vi "format Impedance display.vi"(11 "Imp Value":dbl format="%#_13g") -> (3 "decimal integer string":string)   [LabVIEW 2016, in "CML UI.lvlib"]
doc: "<b>Note:</b> This VI was modified by the <b>Validate DQMH Module</b> tool to turn off automatic error handling."
uses:
  CML UI.lvlib
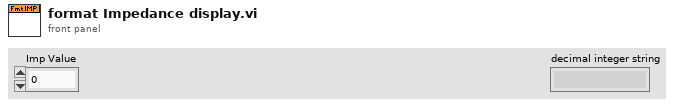
[diagram p1: front panel]
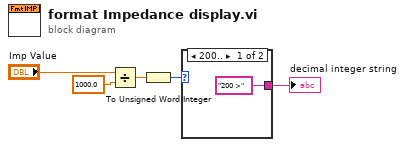
[diagram p0: block diagram]
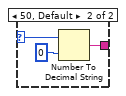
[diagram p2: hidden frame]
diagram:
  n1 = Divide(x="Imp Value", y=1000.0) -> (x/y=w3:dbl)
  n2 = To Unsigned Word Integer(number=w3) -> (unsigned 16bit integer=w2:u16)
  n3 = case shown="200.." w2 {
    selector: w2 -> [_ w8]
    tunnel: ["200 >" w7] -> w1
    frame 200.. {
    }
    frame 50, Default {
      n4 = Number To Decimal String(number=w8, width (-)=i16 0) -> (decimal integer string=w7:string)
    }
  }
  "decimal integer string" <- w1
